vi "半周期测量_有限.vi"() -> ()   [LabVIEW 2013]
uses:
  <userlib>/ArtDAQ/_SubVI/ArtDAQ_CreateCISemiPeriodChan.vi
  <userlib>/ArtDAQ/_SubVI/ArtDAQ_CfgImplicitTiming.vi
  <userlib>/ArtDAQ/_SubVI/ArtDAQ_Read Counter DBL NSamp.vi
panel:
  in  "每通道点数":i32=100
  in  "Stop":bool
  out "数据":dbl[](array[numeric])
  in  "计数器":string="Dev1/ctr0"
  in  "最小测量值":dbl=1e-06 format="%0.6f"
  in  "最大测量值":dbl=10.0 format="%0.6f"
  out "错误输出":errorcluster
  # "通道属性"
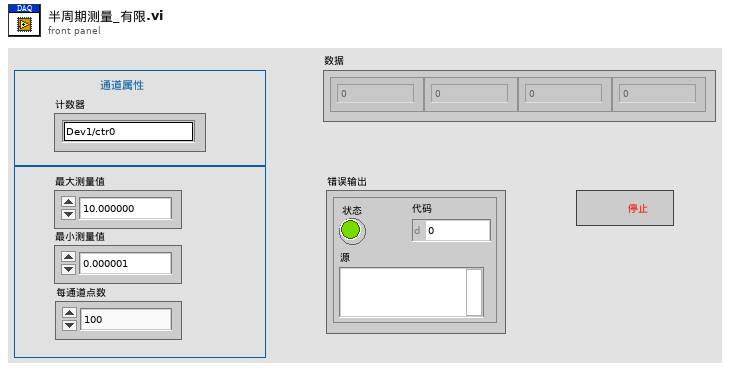
[diagram p1: front panel]
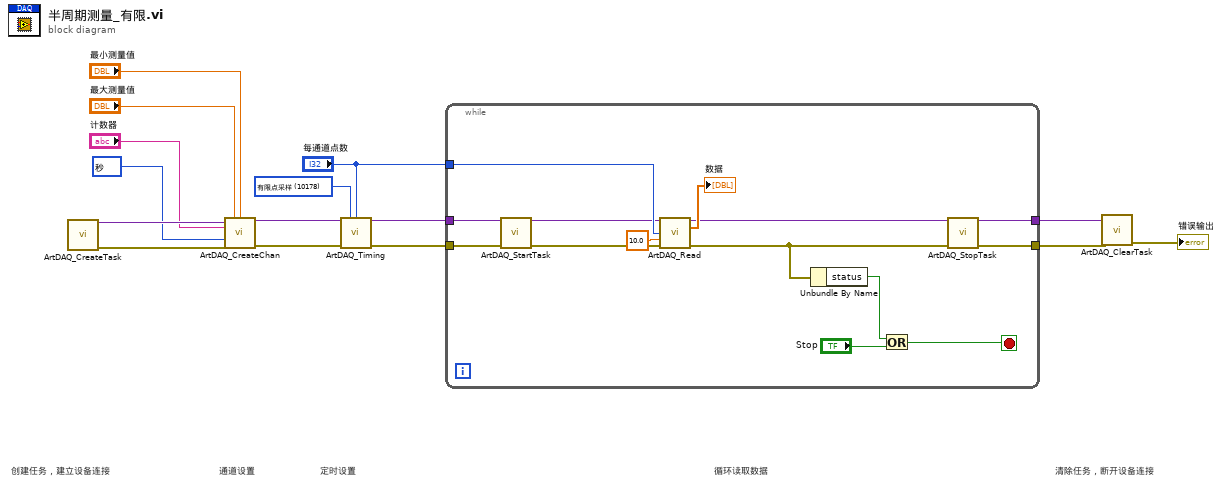
[diagram p0: block diagram]
diagram:
  w4 = 10178 items=["有限点采样"=10178, "连续采样"=10123] ("SampleMode")
  w9 = 10364 items=["秒"=10364, "时钟滴答"=10304, "来自自定义换算"=10065] ("Units")
  # "清除任务，断开设备连接"
  # "循环读取数据"
  # "定时设置"
  # "通道设置"
  # "创建任务，建立设备连接"
  n1 = call <userlib>:"ArtDAQ_CreateTask.vi"() -> ("任务句柄"=w15:variant, "错误输出"=w14:errorcluster)  [unwired: 14 in]
  n2 = call-poly <userlib>:"ArtDAQ_CreateChan.vi"("任务句柄"=w15, "最大值"="最大测量值", "最小值"="最小测量值", "计数器"="计数器", "单位"=w9, "错误输入"=w14) -> ("任务句柄"=w8:variant, "错误输出"=w6:errorcluster)  [unwired: 8 in]
  n3 = call-poly <userlib>:"ArtDAQ_Timing.vi"("任务句柄"=w8, "采样模式"=w4, "每通道采样数"="每通道点数", "错误输入"=w6) -> ("任务句柄"=w7:variant, "错误输出"=w5:errorcluster)  [unwired: 10 in]
  n4 = while {
    tunnel: w7 -> [w29]
    tunnel: w5 -> [w28]
    tunnel: "每通道点数" -> [w27]
    tunnel: [w26] -> w2
    tunnel: [w25] -> w1
    stop <- w16 stop-if-true
    n5 = call <userlib>:"ArtDAQ_StartTask.vi"("任务句柄"=w29, "错误输入"=w28) -> ("任务句柄"=w24:variant, "错误输出"=w23:errorcluster)  [unwired: 12 in]
    n6 = call-poly <userlib>:"ArtDAQ_Read.vi"("任务句柄"=w24, "每通道采样数"=w27, "超时s"=10.0 ("Timeout"), "错误输入"=w23) -> ("任务句柄"=w18:variant, "数据"=→"数据":dbl[], "错误输出"=w17:errorcluster)  [unwired: 8 in, 1 out]
    n7 = Unbundle By Name(w17) -> ("status"=w20:bool)
    n8 = Or(x=w20, y="Stop") -> (x .or. y?=w16:bool)
    n9 = call <userlib>:"ArtDAQ_StopTask.vi"("任务句柄"=w18, "错误输入"=w17) -> ("任务句柄"=w25:variant, "错误输出"=w26:errorcluster)  [unwired: 12 in]
  }
  n10 = call <userlib>:"ArtDAQ_ClearTask.vi"("任务句柄"=w1, "错误输入"=w2) -> ("错误输出"=→"错误输出":errorcluster)  [unwired: 13 in]
